vi "calculations.vi"(8 "error in":errorcluster, 11 "FGV_data":T1) -> (0 "error out":errorcluster, 3 "FGV_data_out":T1)   [LabVIEW 2016]
uses:
  MainFGV/FGV_data.ctl
  TypeDefs/specimen_data.ctl
  TypeDefs/specimen_info.ctl
  <vilib>/Analysis/baseanly.llb/Mean (DBL).vi
  <vilib>/Analysis/NI_AALPro.lvlib
  <vilib>/Analysis/NI_AALBase.lvlib
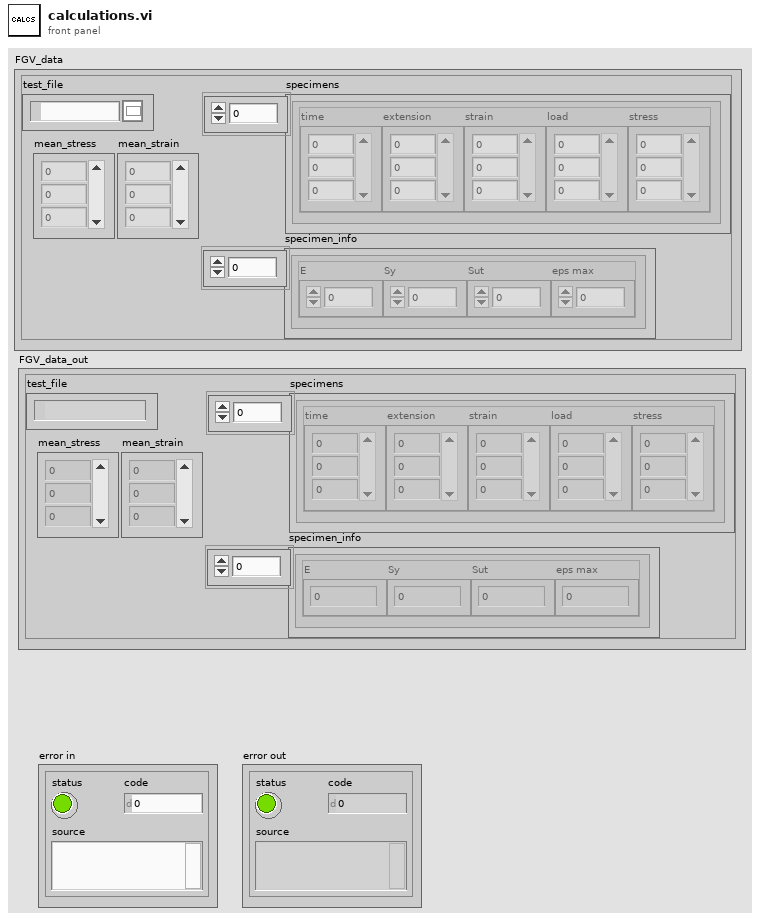
[diagram p1: front panel]
types:
  T1 = typedef "FGV_data.ctl" = cluster{"test_file":path, "specimens":T2[], "mean_strain":dbl[], "mean_stress":dbl[], "specimen_info":T3[]}
  T2 = typedef "specimen_data.ctl" = cluster{"time":dbl[], "extension":dbl[], "strain":dbl[], "load":dbl[], "stress":dbl[]}
  T3 = typedef "specimen_info.ctl" = cluster{"E":dbl, "Sy":dbl, "Sut":dbl, "eps max":dbl}
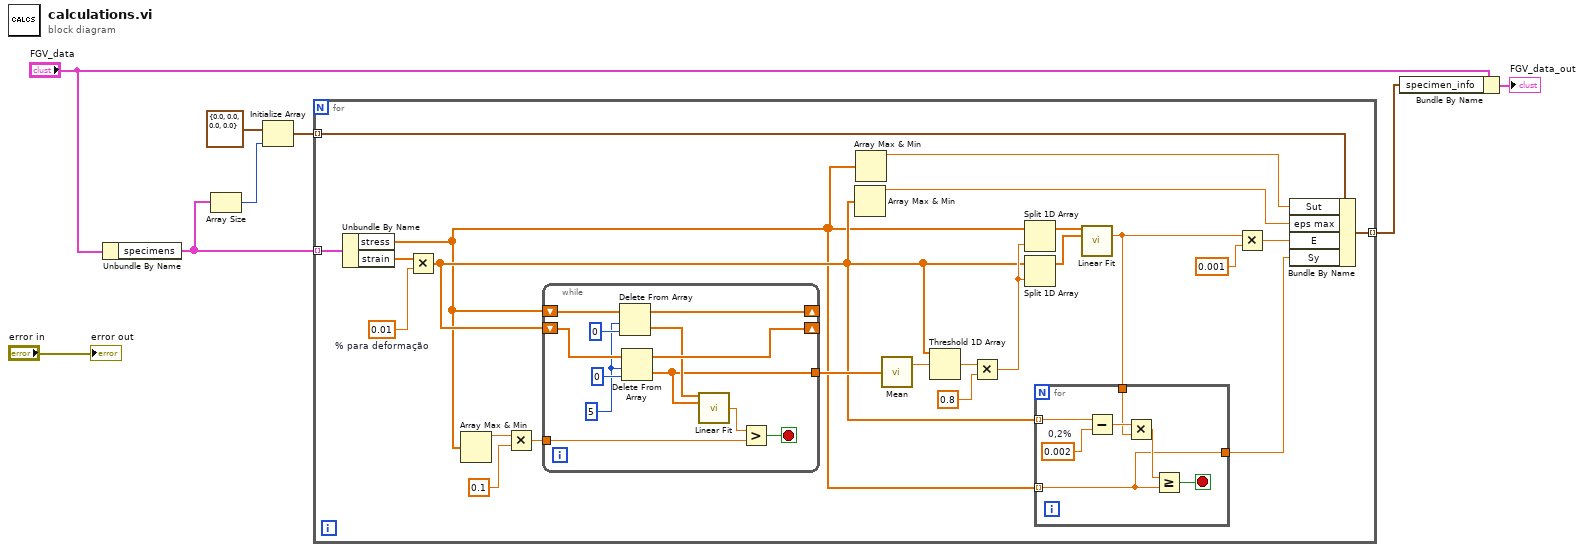
[diagram p0: block diagram]
diagram:
  n1 = Unbundle By Name("FGV_data") -> ("specimens"=w6:T2[])
  n2 = Array Size(array=w6) -> (size(s)=w5:i32)
  n3 = Initialize Array(T3 {"E"=0.0, "Sy"=0.0, "Sut"=0.0, "eps max"=0.0} ("specimen_info"), w5) -> (w4:T3[])
  n4 = for {
    tunnel: w6 -> [w31] mode=indexing
    tunnel: w4 -> [w17] mode=indexing
    tunnel: [w9] -> w2 mode=indexing
    w23 = 0.01  # % para deformação
    n5 = Unbundle By Name(w31) -> ("stress"=w12:dbl[], "strain"=w25:dbl[])
    n6 = Multiply(x=w25, y=w23) -> (x*y=w13:dbl[])
    n7 = Array Max & Min(array=w12) -> (max value=w30:dbl)  [unwired: 3 out]
    n8 = Multiply(x=w30, y=0.1) -> (x*y=w28:dbl)
    n9 = while {
      shift-right: [w45] -> _
      shift-left: w12 -> [w50]
      shift-right: [w46] -> _
      shift-left: w13 -> [w47]
      tunnel: w28 -> [w42]
      tunnel: [w40] -> w27
      stop <- w41 stop-if-true
      w39 = 5 ("length")
      n10 = Delete From Array(array=w50, length=w39, index=0) -> (deleted portion=w44:dbl[], array with subset deleted=w45:dbl[])
      n11 = Delete From Array(array=w47, length=w39, index=0) -> (deleted portion=w40:dbl[], array with subset deleted=w46:dbl[])
      n12 = call <vilib>:"Linear Fit.vi"("Y"=w44, "X"=w40) -> ("intercept"=w43:dbl)  [unwired: 9 in, 4 out]
      n13 = Greater?(x=w43, y=w42) -> (0:w41:bool)
    }
    n14 = Array Max & Min(array=w13) -> (max value=w14:dbl)  [unwired: 3 out]
    n15 = Array Max & Min(array=w12) -> (max value=w15:dbl)  [unwired: 3 out]
    n16 = call-poly <vilib>:"Mean.vi"("X"=w27) -> ("mean"=w26:dbl)  [unwired: 1 out]
    n17 = Threshold 1D Array(2:w26, 3:w13) -> (0:w24:dbl)  [unwired: 1 in]
    n18 = Multiply(x=w24, y=0.8) -> (x*y=w20:dbl)
    n19 = Split 1D Array(array=w12, index=w20) -> (first subarray=w21:dbl[])  [unwired: 1 out]
    n20 = Split 1D Array(array=w13, index=w20) -> (first subarray=w22:dbl[])  [unwired: 1 out]
    n21 = call <vilib>:"Linear Fit.vi"("Y"=w21, "X"=w22) -> ("slope"=w11:dbl)  [unwired: 9 in, 4 out]
    n22 = for {
      tunnel: w13 -> [w38] mode=indexing
      tunnel: w12 -> [w32] mode=indexing
      tunnel: w11 -> [w35]
      tunnel: [w32] -> w10
      stop <- w33 stop-if-true
      w37 = 0.002  # 0,2%
      n23 = Subtract(x=w38, y=w37) -> (x-y=w36:dbl)
      n24 = Multiply(x=w36, y=w35) -> (x*y=w34:dbl)
      n25 = Greater Or Equal?(x=w34, y=w32) -> (x >= y?=w33:bool)
    }
    n26 = Multiply(x=w11, y=0.001) -> (x*y=w16:dbl)
    n27 = Bundle By Name(cluster=w17, "Sut"=w15, "eps max"=w14, "E"=w16, "Sy"=w10) -> (w9:T3)
  }
  n28 = Bundle By Name(cluster="FGV_data", "specimen_info"=w2) -> (→"FGV_data_out":T1)
  "error out" <- "error in"
